vi "ForceTrigger.vi"(8 "error in (no error)":errorcluster, 11 "VISA resource name":refnum<visa-resource-name>) -> (0 "error out":errorcluster, 3 "VISA resource name out":refnum<visa-resource-name>)   [LabVIEW 2009]
uses:
  Packet.ctl
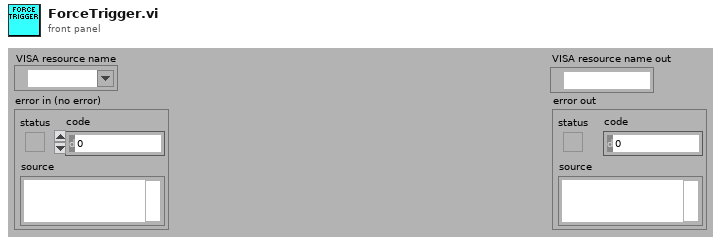
[diagram p1: front panel]
types:
  T1 = typedef "Packet.ctl" = cluster{"Length":u8, "Type":u8, "PID":u8, "Data":u8[], "CRC":u8}
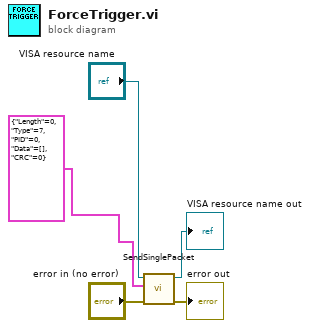
[diagram p0: block diagram]
diagram:
  n1 = call "SendSinglePacket.vi"("error in (no error)"="error in (no error)", "Transmit"=T1 {"Length"=0, "Type"=7, "PID"=0, "Data"=[], "CRC"=0}, "VISA resource name"="VISA resource name") -> ("error out"=→"error out":errorcluster, "VISA resource name out"=→"VISA resource name out":refnum<visa-resource-name>)  [unwired: 6 in, 1 out]
